vi "save_controls.vi"(0 "Array":refnum<vi>[](array[refnum])) -> ()   [LabVIEW 2010]
panel:
  out "Array 2":string[][](array[string])
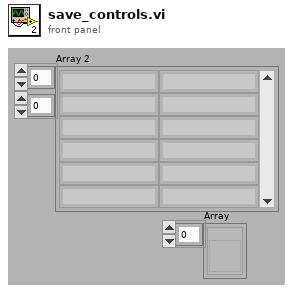
[diagram p1: front panel]
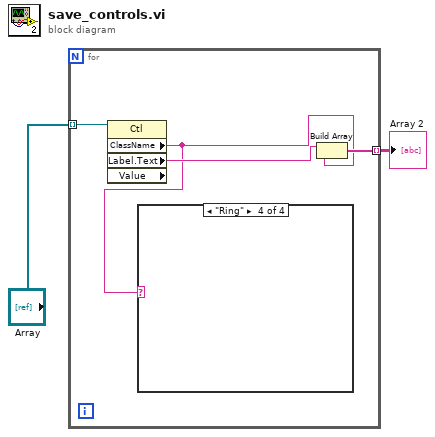
[diagram p0: block diagram]
diagram:
  n1 = for {
    tunnel: "Array" -> [w6] mode=indexing
    tunnel: [w4] -> w1 mode=indexing
    n2 = property class="Ctl" props=["ClassName", "Label", "Text", "Value"](reference=w6) -> ("ClassName"=w3:string, "Label.Text"=w5:string)  [unwired: 1 in, 3 out]
    n3 = case shown="\"Ring\"" w3 {
      frame "Digital", Default {
      }
      frame "String" {
      }
      frame "Boolean" {
      }
      frame "Ring" {
      }
    }
    n4 = Build Array(w5, w3) -> (w4:string[])
  }
  "Array 2" <- w1
